vi "Deconvolution PtByPt (obs 85).vi"(0 "x*y":dbl format="%0.2f", 1 "sample length x*y":i32=100, 2 "y":dbl format="%0.2f", 3 "sample length y":i32=100, 4 "initialize":bool) -> (5 "X":dbl[](array[numeric]), 6 "error":i32)   [LabVIEW 2020, in "NI_PtbyPt.lvlib"]
doc: "Computes the deconvolution of <B>x*y</B> and <B>y</B>."
uses:
  <vilib>/ptbypt/NI_PtbyPt.lvlib
  <vilib>/Analysis/2dsp.llb/Inverse Real FFT.vi
  <vilib>/Analysis/NI_AALPro.lvlib
panel:
  # "This VI is obsolete !!!\nYou should replace this VI in your diagram with the Deconvolution PtByPt VI.\n\nNOTE: Please be aware of that the new Deconvolution PtByPt VI is set to reentrant."
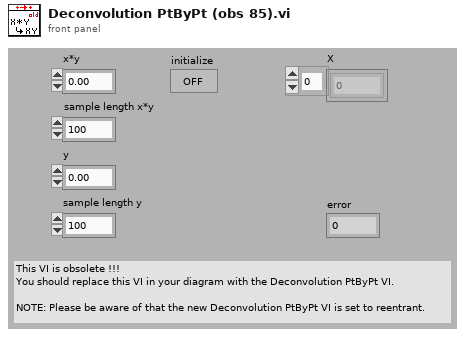
[diagram p1: front panel]
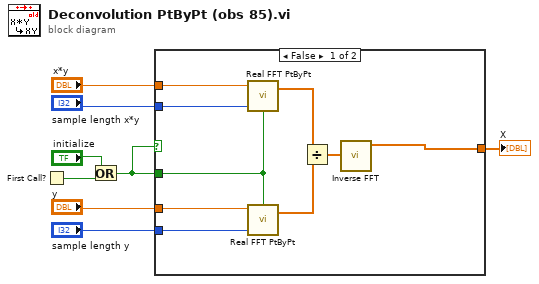
[diagram p0: block diagram]
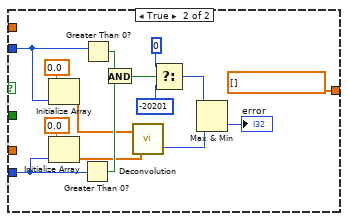
[diagram p2: hidden frame]
diagram:
  n1 = First Call?() -> (First Call?: T/F=w2:bool)
  n2 = Or(x="initialize", y=w2) -> (x .or. y?=w1:bool)
  n3 = case shown="False" w1 {
    tunnel: "x*y" -> [w17 _]
    tunnel: "y" -> [w16 _]
    tunnel: [w12 dbl[] [] ("X")] -> w6
    tunnel: "sample length x*y" -> [w11 w26]
    tunnel: "sample length y" -> [w10 w23]
    tunnel: w1 -> [w9 _]
    frame False {
      n4 = call <vilib>:"Real FFT PtByPt.vi"("initialize"=w9, "sample length"=w11, "x"=w17) -> ("FFT{X}"=w15:cdb[])  [unwired: 1 in, 1 out]
      n5 = call <vilib>:"Real FFT PtByPt.vi"("initialize"=w9, "sample length"=w10, "x"=w16) -> ("FFT{X}"=w14:cdb[])  [unwired: 1 in, 1 out]
      n6 = Divide(x=w15, y=w14) -> (x/y=w13:cdb[])
      n7 = call-poly <vilib>:"Inverse FFT.vi"("FFT {X}"=w13) -> ("X"=w12:dbl[])  [unwired: 9 in, 1 out]
    }
    frame True {
      n8 = Initialize Array(0.0 ("Element Data"), w26) -> (w21:dbl[])
      n9 = Initialize Array(0.0 ("Element Data"), w23) -> (w22:dbl[])
      n10 = Greater Than 0?(x=w23) -> (x > 0?=w29:bool)
      n11 = Greater Than 0?(x=w26) -> (x > 0?=w28:bool)
      n12 = And(x=w28, y=w29) -> (x .and. y?=w30:bool)
      n13 = call <vilib>:"Deconvolution.vi"("Y"=w22, "X * Y"=w21) -> ("error"=w19:i32)  [unwired: 1 out]
      n14 = Select(t=0, s=w30, f=-20201) -> (s? t:f=w20:i32)
      n15 = Max & Min(x=w20, y=w19) -> (min(x,y)=→"error":i32)  [unwired: 1 out]
    }
  }
  "X" <- w6
